vi "Measurement UI.vi"() -> ()   [LabVIEW 2021, in "Frequency Response_Audio ADC_UI.lvlib"]
uses:
  Frequency Response_Audio ADC_UI.lvlib
  shared/Audio ADC Shared.lvlib
panel:
  in  "MeasGraphs":T1(tab)
  out "FrequencyResponseGraph":cluster{"X":dbl[], "Y":dbl[]}(graph) caption="AC"
  out "RMSLevelGraph":cluster{"X":dbl[], "Y":dbl[]}(graph) caption="AC"
  out "THDResponseGraph":cluster{"X":dbl[], "Y":dbl[]}(graph) caption="AC"
  out "THD+NResponseGraph":cluster{"X":dbl[], "Y":dbl[]}(graph) caption="AC"
  out "TimeDomainGraph":cluster{dbl, "dt":dbl, "Time domain":dbl[]}[](graph) caption="AC"
  in  "Bit clock edge sync":u32=1
  in  "Frame sync pulse width":u32=32
  in  "Frame length":u32=64
  in  "Data justification":u32 caption="Data Justification"
  in  "Endianness":u32
  in  "Channel 0 offset":u32=1
  in  "Bit depth":u32=24
  in  "Channel length":u32=32
  in  "Channel count per frame":u32=2
  in  "Frame sync edge for channel 0":u32=1
  out "Time domain plot sizes":i32[](array[numeric])
  out "THD+N response":dbl[](array[numeric])
  out "Frequency response":dbl[](array[numeric])
  out "Time domain":dbl[](array[numeric])
  out "dt":dbl
  out "RMS levels":dbl[](array[numeric])
  out "THD response":dbl[](array[numeric])
  out "Frequency steps":dbl[](array[numeric])
  in  "Configure Protocol Settings":bool
  in  "Analog source resource name":string(combo) caption="RESOURCE NAME"
  in  "Protocol capture resource name":string(combo) caption="RESOURCE NAME"
  in  "Data line":u32 caption="DATA LINE"
  in  "Channel":u32 caption="CHANNEL"
  in  "MeasSettingsOptions":i32(listbox)=-1
  in  "Settling time":dbl caption="SETTLING TIME" format="%#_6ps"
  in  "Settling cycles":i32 caption="SETTLING CYCLES"
  in  "Maximum harmonic":i32=5 caption="MAX HARMONIC"
  in  "DC Offset":dbl caption="DC OFFSET" format="%#_6pV"
  out "Protocol settings":string="Protocol settings"
  in  "Sample rate":dbl=44100.0 caption="SAMPLE RATE" format="%#.6pHz"
  in  "Frequency spacing":string(combo)="Logarithmic" caption="FREQUENCY SPACING"
  in  "Measurement duration":dbl=0.001 caption="MEASUREMENT DURATION" format="%#_6ps"
  in  "Measurement cycles":i32=10 caption="MEASUREMENT CYCLES"
  in  "Frequency steps":i32=20 caption="FREQUENCY STEPS"
  out "Analog source":string="Analog source "
  in  "Amplitude":dbl=-1.0 caption="AMPLITUDE" format="%#_6pdB"
  in  "Full scale range":dbl=2.825 caption="FULL SCALE RANGE" format="%.3pV"
  in  "Frequency stop":dbl=10000.0 caption="FREQUENCY STOP" format="%#_6pHz"
  in  "Frequency start":dbl=100.0 caption="FREQUENCY START" format="%#_6pHz"
  out "Measurement settings":string="Measurement settings"
  in  "MeasSettings":bool
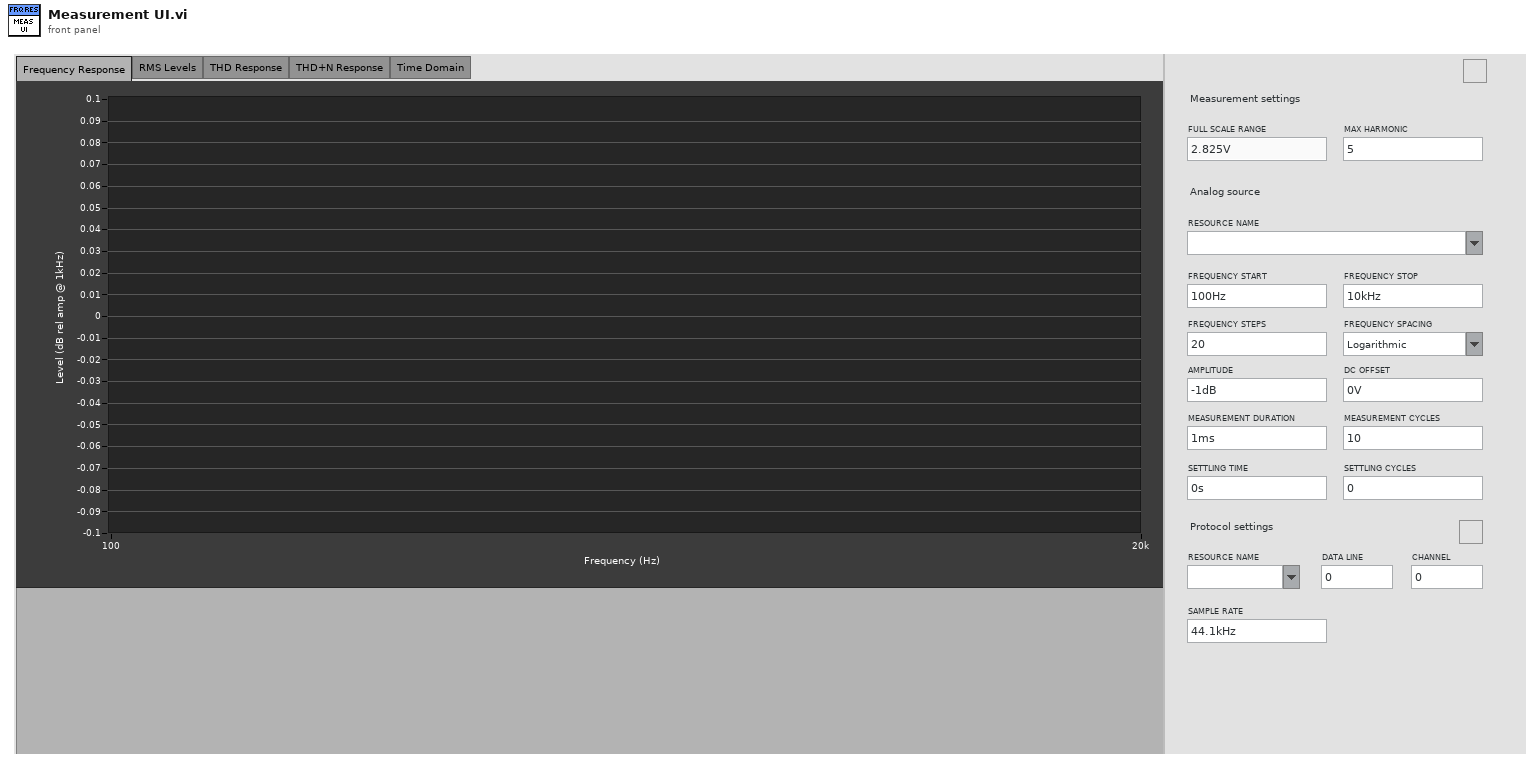
[diagram p1: front panel]
types:
  T1 = enum32{"Frequency Response", "RMS Levels", "THD Response", "THD+N Response", "Time Domain", "Hidden Controls"}
  T2 = enum16{"open", "replace", "create", "open or create", "replace or create", "replace or create with confirmation"}
  T3 = typedef "PDM Shared.lvlib/PCM Frame Sync Control.ctl" = cluster{"Frame Length":u16, "Frame Sync Pulse Width":u16, "Bit Clock Edge  Sync":T4}
  T4 = typedef "PDM Shared.lvlib/Digital Edge.ctl" = enum8{"Rising", "Falling"}
  T5 = typedef "PDM Shared.lvlib/PCM Data Format Configuration.ctl" = cluster{"Frame Sync Edge for Channel 0":T4, "Channel Count Per Frame":u8, "Channel Length":u16, "Bit Depth":u8, "Channel 0 Offset":u16, "Endianness":T6, "Data Justification":T7}
  T6 = typedef "PDM Shared.lvlib/PCM Bit Endianness.ctl" = enum16{"MSB First", "LSB First"}
  T7 = typedef "PDM Shared.lvlib/PCM Data Justification.ctl" = enum16{"Left Justified", "Right Justified"}
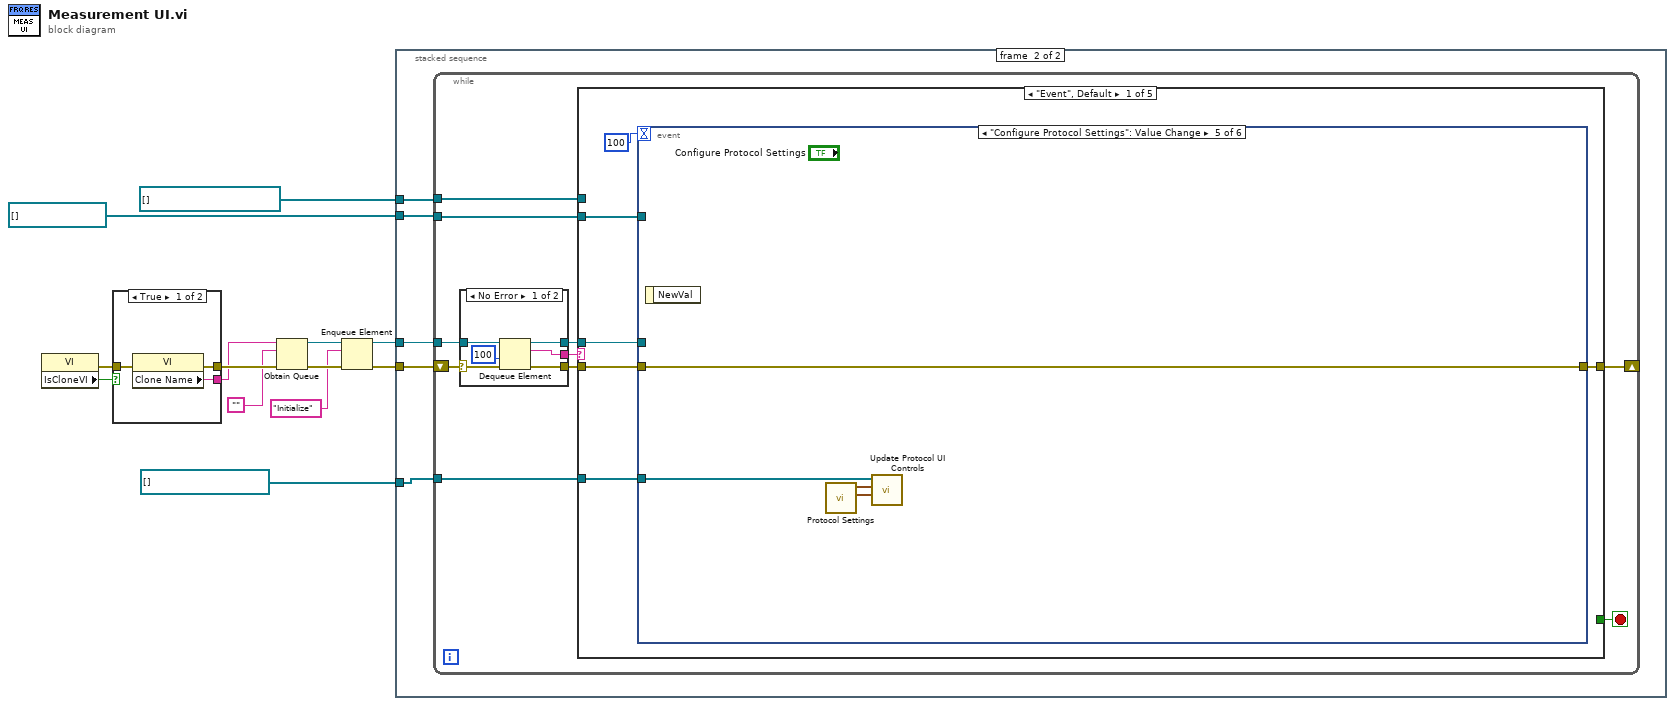
[diagram p0: block diagram]
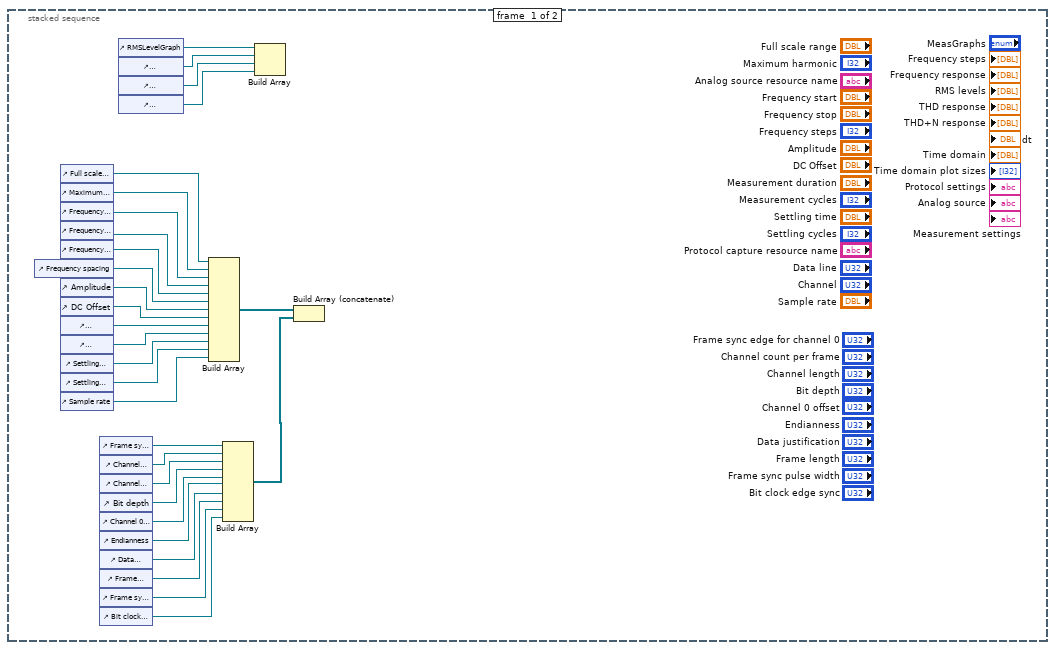
[diagram p2: hidden frame]
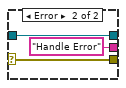
[diagram p3: hidden frame]
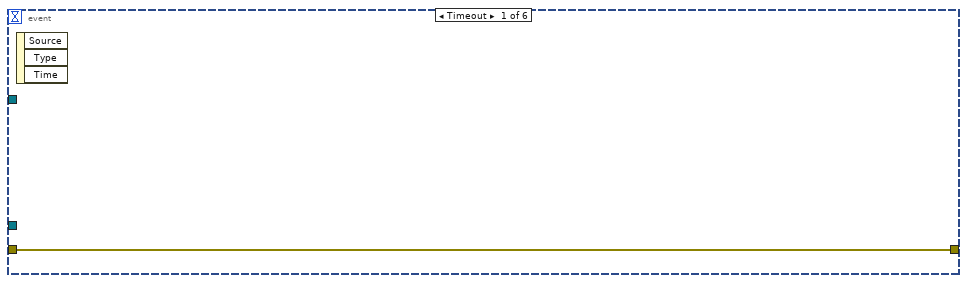
[diagram p4: hidden frame]
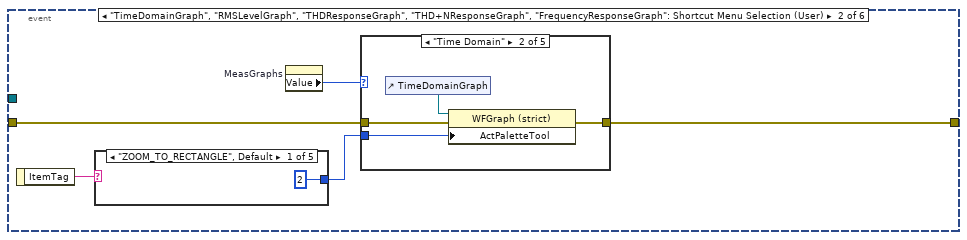
[diagram p5: hidden frame]
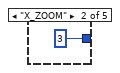
[diagram p6: hidden frame]
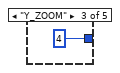
[diagram p7: hidden frame]
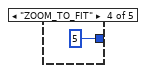
[diagram p8: hidden frame]
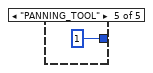
[diagram p9: hidden frame]
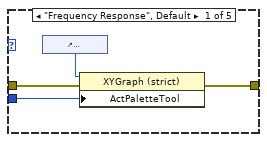
[diagram p10: hidden frame]
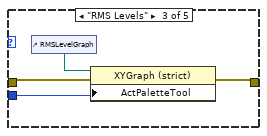
[diagram p11: hidden frame]
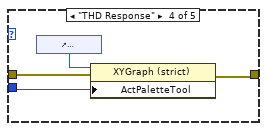
[diagram p12: hidden frame]
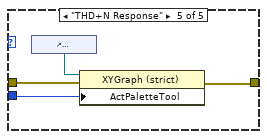
[diagram p13: hidden frame]
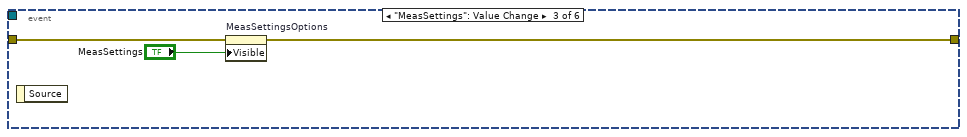
[diagram p14: hidden frame]
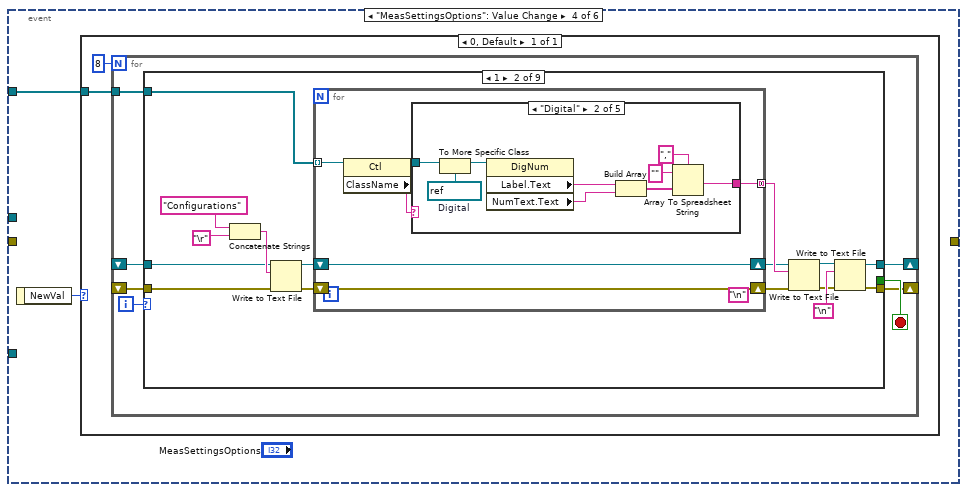
[diagram p15: hidden frame]
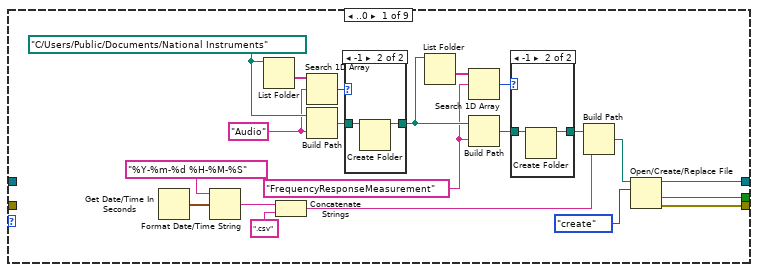
[diagram p16: hidden frame]
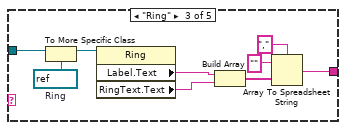
[diagram p20: hidden frame]
diagram:
  n1 = property class="VI"() -> (error out=w4:errorcluster, "IsCloneVI"=w5:bool)  [unwired: 2 in, 1 out]
  n2 = case shown="True" w5 {
    tunnel: [w16 w19] -> w13
    tunnel: [w15 w18] -> w12
    tunnel: w4 -> [w14 w17]
    frame True {
      n3 = property class="VI"(error in=w14) -> (error out=w16:errorcluster, "Clone Name"=w15:string)  [unwired: 1 in, 1 out]
    }
    frame False {
      n4 = property class="VI"(error in=w17) -> (error out=w19:errorcluster, "Name"=w18:string)  [unwired: 1 in, 1 out]
    }
  }
  n5 = Obtain Queue(name (unnamed)=w12, element data type="", error in (no error)=w13) -> (queue out=w9:refnum<queue>, error out=w11:errorcluster)  [unwired: 2 in, 1 out]
  n6 = Enqueue Element(queue=w9, element="Initialize", error in (no error)=w11) -> (queue out=w8:refnum<queue>, error out=w10:errorcluster)  [unwired: 1 in, 1 out]
  n7 = stacked-sequence {
    tunnel: w10 -> [_ w53]
    tunnel: w8 -> [_ w52]
    tunnel: refnum<vi>[] [] -> [_ w51]
    tunnel: refnum<vi>[] [] -> [_ w50]
    tunnel: refnum<vi>[] [] -> [_ w49]
    frame #0 {
      n8 = control-ref of="Frequency spacing"() -> (w43:refnum<vi>)
      n9 = control-ref of="Full scale range"() -> (w48:refnum<vi>)
      n10 = control-ref of="Maximum harmonic"() -> (w47:refnum<vi>)
      n11 = control-ref of="Frequency start"() -> (w46:refnum<vi>)
      n12 = control-ref of="Frequency stop"() -> (w45:refnum<vi>)
      n13 = control-ref of="Frequency steps"() -> (w44:refnum<vi>)
      n14 = control-ref of="Amplitude"() -> (w37:refnum<vi>)
      n15 = control-ref of="DC Offset"() -> (w36:refnum<vi>)
      n16 = control-ref of="Measurement duration"() -> (w42:refnum<vi>)
      n17 = control-ref of="Measurement cycles"() -> (w41:refnum<vi>)
      n18 = control-ref of="Settling time"() -> (w40:refnum<vi>)
      n19 = control-ref of="Settling cycles"() -> (w39:refnum<vi>)
      n20 = control-ref of="Sample rate"() -> (w38:refnum<vi>)
      n21 = control-ref of="Frame sync edge for channel 0"() -> (w31:refnum<vi>)
      n22 = control-ref of="Channel count per frame"() -> (w30:refnum<vi>)
      n23 = control-ref of="Channel length"() -> (w29:refnum<vi>)
      n24 = control-ref of="Bit depth"() -> (w28:refnum<vi>)
      n25 = control-ref of="Channel 0 offset"() -> (w27:refnum<vi>)
      n26 = control-ref of="Endianness"() -> (w26:refnum<vi>)
      n27 = control-ref of="Data justification"() -> (w25:refnum<vi>)
      n28 = control-ref of="Frame length"() -> (w24:refnum<vi>)
      n29 = control-ref of="Frame sync pulse width"() -> (w23:refnum<vi>)
      n30 = control-ref of="Bit clock edge sync"() -> (w22:refnum<vi>)
      n31 = control-ref of="RMSLevelGraph"() -> (w35:refnum<vi>)
      n32 = control-ref of="THDResponseGraph"() -> (w34:refnum<vi>)
      n33 = control-ref of="THD+NResponseGraph"() -> (w33:refnum<vi>)
      n34 = control-ref of="FrequencyResponseGraph"() -> (w32:refnum<vi>)
      n35 = Build Array(w48, w47, w46, w45, w44, w43, w37, w36, w42, w41, w40, w39, w38) -> (w21:refnum<vi>[])
      n36 = Build Array(w31, w30, w29, w28, w27, w26, w25, w24, w23, w22) -> (w20:refnum<vi>[])
      n37 = Build Array(w35, w34, w33, w32) -> ()  [unwired: 1 out]
      n38 = Build Array (concatenate)(w21, w20) -> ()  [unwired: 1 out]
    }
    frame #1 {
      n39 = while {
        shift-right: [w58] -> _
        shift-left: w53 -> [w63]
        tunnel: w52 -> [w61]
        tunnel: w49 -> [w56]
        tunnel: w51 -> [w55]
        tunnel: w50 -> [w54]
        stop <- w57 stop-if-true
        n40 = case shown="No Error" w63 {
          selector: w63 -> [w69 w72]
          tunnel: [w68 w72] -> w62
          tunnel: w61 -> [w67 w71]
          tunnel: [w66 w71] -> w60
          tunnel: [w65 "Handle Error"] -> w59
          frame No Error {
            n41 = Dequeue Element(queue=w67, timeout in ms (-1)=100, error in (no error)=w69) -> (queue out=w66:refnum<queue>, element=w65:string, error out=w68:errorcluster)  [unwired: 1 out]
          }
          frame Error {
          }
        }
        n42 = case shown="\"Event\", Default" w59 {
          tunnel: w62 -> [w77 w395 w432 w459 w460]
          tunnel: w60 -> [w75 _ _ w457 _]
          tunnel: [w78 w395 w432 w454 w460] -> w58
          tunnel: [_ _ _ TRUE _] -> w57
          tunnel: w56 -> [_ _ w406 _ _]
          tunnel: w55 -> [w74 _ _ _ _]
          tunnel: w54 -> [w73 _ _ _ _]
          frame "Event", Default {
            n43 = event shown="[4] \"Configure Protocol Settings\": Value Change" {
              selector: _ -> [_ _ _ _ _ _]
              dyn-events: _ -> [_ _ _ _ _ _]
              timeout: 100 -> [_ _ _ _ _ _]
              tunnel: [w79 w80 w110 _ w382 w385] -> w78
              tunnel: w77 -> [w79 w82 w112 _ w382 w386]
              tunnel: w75 -> [_ _ _ _ _ w384]
              tunnel: w74 -> [_ _ _ _ w379 _]
              tunnel: w73 -> [_ _ _ w113 _ _]
              event Timeout {
                n44 = event-data() -> ()  [unwired: 1 in, 3 out]
              }
              event "TimeDomainGraph", "RMSLevelGraph", "THDResponseGraph", "THD+NResponseGraph", "FrequencyResponseGraph": Shortcut Menu Selection (User) {
                n45 = event-data() -> ("ItemTag"=w83:string)  [unwired: 1 in]
                n46 = case shown="\"ZOOM_TO_RECTANGLE\", Default" w83 {
                  tunnel: [2 3 4 5 1] -> w81
                  frame "ZOOM_TO_RECTANGLE", Default {
                  }
                  frame "X_ZOOM" {
                  }
                  frame "Y_ZOOM" {
                  }
                  frame "ZOOM_TO_FIT" {
                  }
                  frame "PANNING_TOOL" {
                  }
                }
                n47 = property on="MeasGraphs" class="TabCtl (strict)"() -> ("Value"=w84:T1)  [unwired: 2 in, 2 out]
                n48 = case shown="\"Time Domain\"" w84 {
                  tunnel: w82 -> [w93 w96 w100 w105 w109]
                  tunnel: w81 -> [w90 w95 w99 w102 w108]
                  tunnel: [w92 w94 w98 w104 w107] -> w80
                  frame "Frequency Response", Default {
                    n49 = control-ref of="FrequencyResponseGraph"() -> (w91:refnum<vi>)
                    n50 = property class="XYGraph (strict)"(reference=w91, error in=w93, "ActPaletteTool"=w90) -> (error out=w92:errorcluster)  [unwired: 1 out]
                  }
                  frame "Time Domain" {
                    n51 = control-ref of="TimeDomainGraph"() -> (w97:refnum<vi>)
                    n52 = property class="WFGraph (strict)"(reference=w97, error in=w96, "ActPaletteTool"=w95) -> (error out=w94:errorcluster)  [unwired: 1 out]
                  }
                  frame "RMS Levels" {
                    n53 = control-ref of="RMSLevelGraph"() -> (w101:refnum<vi>)
                    n54 = property class="XYGraph (strict)"(reference=w101, error in=w100, "ActPaletteTool"=w99) -> (error out=w98:errorcluster)  [unwired: 1 out]
                  }
                  frame "THD Response" {
                    n55 = control-ref of="THDResponseGraph"() -> (w103:refnum<vi>)
                    n56 = property class="XYGraph (strict)"(reference=w103, error in=w105, "ActPaletteTool"=w102) -> (error out=w104:errorcluster)  [unwired: 1 out]
                  }
                  frame "THD+N Response" {
                    n57 = control-ref of="THD+NResponseGraph"() -> (w106:refnum<vi>)
                    n58 = property class="XYGraph (strict)"(reference=w106, error in=w109, "ActPaletteTool"=w108) -> (error out=w107:errorcluster)  [unwired: 1 out]
                  }
                }
              }
              event "MeasSettings": Value Change {
                n59 = event-data() -> ()  [unwired: 1 in, 1 out]
                n60 = property on="MeasSettingsOptions" class="LstBox (strict)"(error in=w112, "Visible"="MeasSettings") -> (error out=w110:errorcluster)  [unwired: 1 in, 1 out]
              }
              event "MeasSettingsOptions": Value Change {
                n61 = event-data() -> ("NewVal"=w114:i32)  [unwired: 1 in]
                n62 = case shown="0, Default" w114 {
                  tunnel: w113 -> [w115]
                  frame 0, Default {
                    n63 = for {
                      N: 8 -> [_]
                      shift-right: [w121] -> _
                      shift-left: _ -> [w120]
                      shift-right: [w119] -> _
                      shift-left: _ -> [w118]
                      tunnel: w115 -> [w117]
                      i -> [w123]
                      stop <- w122 stop-if-true
                      n64 = case shown="1" w123 {
                        tunnel: [w137 _ _ _ _ _ _ _ _] -> w122
                        tunnel: [w143 w152 w216 w247 w279 w311 w341 refnum<file> refnum ("refnum out") w378] -> w121
                        tunnel: w120 -> [_ w163 w236 w268 w300 w332 w349 w376 w378]
                        tunnel: [w136 w153 w214 w245 w277 w309 w340 w374 w377] -> w119
                        tunnel: w118 -> [_ w161 w235 w267 w299 w331 w350 w373 w377]
                        tunnel: w117 -> [_ w151 _ _ _ _ _ _ _]
                        frame ..0 {
                          w132 = "FrequencyResponseMeasurement" ("prompt")
                          w139 = "Audio" ("prompt")
                          w142 = path "C:/Users/Public/Documents/National Instruments" ("base path")
                          n65 = Get Date/Time In Seconds() -> (seconds since 1Jan1904=w129:timestamp)
                          n66 = Format Date/Time String(time format string (%c)="%Y-%m-%d %H-%M-%S", seconds (now)=w129) -> (date/time string=w128:string)  [unwired: 1 in]
                          n67 = List Folder(path=w142) -> (folder names=w140:string[])  [unwired: 3 in, 3 out]
                          n68 = Concatenate Strings(w128, ".csv" ("string")) -> (w125:string)
                          n69 = Search 1D Array(1D array=w140, element=w139) -> (index of element=w138:i32)  [unwired: 1 in]
                          n70 = Build Path(base path=w142, name or relative path=w139) -> (appended path=w141:path)
                          n71 = case shown="-1" w138 {
                            tunnel: w141 -> [w148 w150]
                            tunnel: [w148 w149] -> w133
                            frame Default {
                            }
                            frame -1 {
                              n72 = Create Folder(path (use dialog)=w150) -> (created path=w149:path)  [unwired: 2 in, 2 out]
                            }
                          }
                          n73 = List Folder(path=w133) -> (folder names=w135:string[])  [unwired: 3 in, 3 out]
                          n74 = Search 1D Array(1D array=w135, element=w132) -> (index of element=w134:i32)  [unwired: 1 in]
                          n75 = Build Path(base path=w133, name or relative path=w132) -> (appended path=w131:path)
                          n76 = case shown="-1" w134 {
                            tunnel: w131 -> [w145 w147]
                            tunnel: [w145 w146] -> w126
                            frame Default {
                            }
                            frame -1 {
                              n77 = Create Folder(path (use dialog)=w147) -> (created path=w146:path)  [unwired: 2 in, 2 out]
                            }
                          }
                          n78 = Build Path(base path=w126, name or relative path=w125) -> (appended path=w124:path)
                          n79 = Open/Create/Replace File(file path (use dialog)=w124, operation (0:open)=T2."create") -> (refnum out=w143:refnum<file>, cancelled=w137:bool, error out=w136:errorcluster)  [unwired: 4 in]
                        }
                        frame 1 {
                          (unwired) "\n"
                          n80 = Concatenate Strings("Configurations" ("format string"), "\r") -> (w164:string)
                          n81 = Write to Text File(file (use dialog)=w163, text=w164, error in=w161) -> (refnum out=w160:refnum<file>, error out=w162:errorcluster)  [unwired: 1 in, 1 out]
                          n82 = for {
                            shift-right: [w172] -> w158
                            shift-left: w160 -> [w172]
                            shift-right: [w171] -> w157
                            shift-left: w162 -> [w171]
                            tunnel: [w170] -> w159 mode=concatenating
                            tunnel: w151 -> [w167] mode=indexing
                            n83 = property class="Ctl"(reference=w167) -> (reference out=w169:refnum<vi>, "ClassName"=w168:string)  [unwired: 1 in, 1 out]
                            n84 = case shown="\"Digital\"" w168 {
                              tunnel: [_ w176 w186 w195 w204] -> w170
                              tunnel: w169 -> [_ w174 w184 w199 w208]
                              frame Default {
                              }
                              frame "Digital" {
                                w173 = refnum<vi> refnum  # Digital
                                n85 = To More Specific Class(target class=w173, reference=w174) -> (specific class reference=w175:refnum<vi>)  [unwired: 1 in, 1 out]
                                n86 = property class="DigNum"(reference=w175) -> ("Label.Text"=w181:string, "NumText.Text"=w180:string)  [unwired: 1 in, 2 out]
                                n87 = Build Array(w181, w180) -> (w177:string[])
                                n88 = Array To Spreadsheet String(delimiter (Tab)=",", array=w177, 3:"" ("format string")) -> (spreadsheet string=w176:string)
                              }
                              frame "Ring" {
                                w183 = refnum<vi> refnum  # Ring
                                n89 = To More Specific Class(target class=w183, reference=w184) -> (specific class reference=w185:refnum<vi>)  [unwired: 1 in, 1 out]
                                n90 = property class="Ring"(reference=w185) -> ("Label.Text"=w182:string, "RingText.Text"=w190:string)  [unwired: 1 in, 2 out]
                                n91 = Build Array(w182, w190) -> (w187:string[])
                                n92 = Array To Spreadsheet String(delimiter (Tab)=",", array=w187, 3:"" ("format string")) -> (spreadsheet string=w186:string)
                              }
                              frame "Enum" {
                                w198 = refnum<vi> refnum  # Enum
                                n93 = To More Specific Class(target class=w198, reference=w199) -> (specific class reference=w194:refnum<vi>)  [unwired: 1 in, 1 out]
                                n94 = property class="Enum"(reference=w194) -> ("Label.Text"=w193:string, "RingText.Text"=w192:string)  [unwired: 1 in, 2 out]
                                n95 = Build Array(w193, w192) -> (w191:string[])
                                n96 = Array To Spreadsheet String(delimiter (Tab)=",", array=w191, 3:"" ("format string")) -> (spreadsheet string=w195:string)
                              }
                              frame "ComboBox" {
                                w207 = refnum<vi> refnum  # ComboBox
                                n97 = To More Specific Class(target class=w207, reference=w208) -> (specific class reference=w203:refnum<vi>)  [unwired: 1 in, 1 out]
                                n98 = property class="CmbBox"(reference=w203) -> ("Label.Text"=w202:string, "Value"=w201:string)  [unwired: 1 in, 2 out]
                                n99 = Build Array(w202, w201) -> (w200:string[])
                                n100 = Array To Spreadsheet String(delimiter (Tab)=",", array=w200, 3:"" ("format string")) -> (spreadsheet string=w204:string)
                              }
                            }
                          }
                          n101 = Write to Text File(file (use dialog)=w158, text=w159, error in=w157) -> (refnum out=w155:refnum<file>, error out=w154:errorcluster)  [unwired: 1 in, 1 out]
                          n102 = Write to Text File(file (use dialog)=w155, text="\n", error in=w154) -> (refnum out=w152:refnum<file>, error out=w153:errorcluster)  [unwired: 1 in, 1 out]
                        }
                        frame 2 {
                          w209 = "\r"
                          n103 = property on="FrequencyResponseGraph" class="XYGraph (strict)"() -> ("Value"=w211:cluster{"X":dbl[], "Y":dbl[]})  [unwired: 2 in, 2 out]
                          n104 = Concatenate Strings("Results" ("string"), w209, "Frequency Response" ("string"), w209) -> (w233:string)
                          n105 = Write to Text File(file (use dialog)=w236, text=w233, error in=w235) -> (refnum out=w229:refnum<file>, error out=w228:errorcluster)  [unwired: 1 in, 1 out]
                          n106 = Build Array("Frequency (Hz)", "Level (dB rel amp @ 1kHz)") -> (w232:string[])
                          n107 = Unbundle By Name(w211) -> ("X"=w220:dbl[], "Y"=w221:dbl[])
                          n108 = Array To Spreadsheet String(delimiter (Tab)=",", array=w232, 3:"" ("format string")) -> (spreadsheet string=w227:string)
                          n109 = for {
                            tunnel: w220 -> [w241] mode=indexing
                            tunnel: w221 -> [w237] mode=indexing
                            tunnel: [w238] -> w222 mode=indexing
                            n110 = Format Into String(w241) -> (resulting string=w239:string)  [unwired: 3 in, 1 out]
                            n111 = Format Into String(w237) -> (resulting string=w240:string)  [unwired: 3 in, 1 out]
                            n112 = Build Array(w239, w240) -> (w238:string[])
                          }
                          n113 = Write to Text File(file (use dialog)=w229, text=w227, error in=w228) -> (refnum out=w226:refnum<file>, error out=w225:errorcluster)  [unwired: 1 in, 1 out]
                          n114 = Array To Spreadsheet String(delimiter (Tab)=",", array=w222, 3:"" ("format string")) -> (spreadsheet string=w219:string)
                          n115 = Write to Text File(file (use dialog)=w226, text=w219, error in=w225) -> (refnum out=w218:refnum<file>, error out=w217:errorcluster)  [unwired: 1 in, 1 out]
                          n116 = Write to Text File(file (use dialog)=w218, text="\n", error in=w217) -> (refnum out=w216:refnum<file>, error out=w214:errorcluster)  [unwired: 1 in, 1 out]
                        }
                        frame 3 {
                          n117 = property on="RMSLevelGraph" class="XYGraph (strict)"() -> ("Value"=w242:cluster{"X":dbl[], "Y":dbl[]})  [unwired: 2 in, 2 out]
                          n118 = Concatenate Strings("RMS Level" ("string"), "\r") -> (w265:string)
                          n119 = Build Array("Frequency (Hz)", "Level (Vrms)") -> (w264:string[])
                          n120 = Write to Text File(file (use dialog)=w268, text=w265, error in=w267) -> (refnum out=w261:refnum<file>, error out=w260:errorcluster)  [unwired: 1 in, 1 out]
                          n121 = Array To Spreadsheet String(delimiter (Tab)=",", array=w264, 3:"" ("format string")) -> (spreadsheet string=w259:string)
                          n122 = Unbundle By Name(w242) -> ("X"=w252:dbl[], "Y"=w253:dbl[])
                          n123 = Write to Text File(file (use dialog)=w261, text=w259, error in=w260) -> (refnum out=w258:refnum<file>, error out=w257:errorcluster)  [unwired: 1 in, 1 out]
                          n124 = for {
                            tunnel: w252 -> [w273] mode=indexing
                            tunnel: w253 -> [w269] mode=indexing
                            tunnel: [w270] -> w254 mode=indexing
                            n125 = Format Into String(w273) -> (resulting string=w271:string)  [unwired: 3 in, 1 out]
                            n126 = Format Into String(w269) -> (resulting string=w272:string)  [unwired: 3 in, 1 out]
                            n127 = Build Array(w271, w272) -> (w270:string[])
                          }
                          n128 = Array To Spreadsheet String(delimiter (Tab)=",", array=w254, 3:"" ("format string")) -> (spreadsheet string=w251:string)
                          n129 = Write to Text File(file (use dialog)=w258, text=w251, error in=w257) -> (refnum out=w249:refnum<file>, error out=w248:errorcluster)  [unwired: 1 in, 1 out]
                          n130 = Write to Text File(file (use dialog)=w249, text="\n", error in=w248) -> (refnum out=w247:refnum<file>, error out=w245:errorcluster)  [unwired: 1 in, 1 out]
                        }
                        frame 4 {
                          n131 = Concatenate Strings("THD Response" ("string"), "\r") -> (w297:string)
                          n132 = property on="THDResponseGraph" class="XYGraph (strict)"() -> ("Value"=w274:cluster{"X":dbl[], "Y":dbl[]})  [unwired: 2 in, 2 out]
                          n133 = Build Array("Frequency (Hz)", "THD (dB)") -> (w296:string[])
                          n134 = Write to Text File(file (use dialog)=w300, text=w297, error in=w299) -> (refnum out=w293:refnum<file>, error out=w292:errorcluster)  [unwired: 1 in, 1 out]
                          n135 = Array To Spreadsheet String(delimiter (Tab)=",", array=w296, 3:"" ("format string")) -> (spreadsheet string=w291:string)
                          n136 = Unbundle By Name(w274) -> ("X"=w284:dbl[], "Y"=w285:dbl[])
                          n137 = Write to Text File(file (use dialog)=w293, text=w291, error in=w292) -> (refnum out=w290:refnum<file>, error out=w289:errorcluster)  [unwired: 1 in, 1 out]
                          n138 = for {
                            tunnel: w284 -> [w305] mode=indexing
                            tunnel: w285 -> [w301] mode=indexing
                            tunnel: [w302] -> w286 mode=indexing
                            n139 = Format Into String(w305) -> (resulting string=w303:string)  [unwired: 3 in, 1 out]
                            n140 = Format Into String(w301) -> (resulting string=w304:string)  [unwired: 3 in, 1 out]
                            n141 = Build Array(w303, w304) -> (w302:string[])
                          }
                          n142 = Array To Spreadsheet String(delimiter (Tab)=",", array=w286, 3:"" ("format string")) -> (spreadsheet string=w283:string)
                          n143 = Write to Text File(file (use dialog)=w290, text=w283, error in=w289) -> (refnum out=w281:refnum<file>, error out=w280:errorcluster)  [unwired: 1 in, 1 out]
                          n144 = Write to Text File(file (use dialog)=w281, text="\n", error in=w280) -> (refnum out=w279:refnum<file>, error out=w277:errorcluster)  [unwired: 1 in, 1 out]
                        }
                        frame 5 {
                          n145 = property on="THD+NResponseGraph" class="XYGraph (strict)"() -> ("Value"=w306:cluster{"X":dbl[], "Y":dbl[]})  [unwired: 2 in, 2 out]
                          n146 = Concatenate Strings("THD+N Response" ("string"), "\r") -> (w329:string)
                          n147 = Build Array("Frequency (Hz)", "THD+N (dB)") -> (w328:string[])
                          n148 = Write to Text File(file (use dialog)=w332, text=w329, error in=w331) -> (refnum out=w325:refnum<file>, error out=w324:errorcluster)  [unwired: 1 in, 1 out]
                          n149 = Array To Spreadsheet String(delimiter (Tab)=",", array=w328, 3:"" ("format string")) -> (spreadsheet string=w323:string)
                          n150 = Unbundle By Name(w306) -> ("X"=w316:dbl[], "Y"=w317:dbl[])
                          n151 = Write to Text File(file (use dialog)=w325, text=w323, error in=w324) -> (refnum out=w322:refnum<file>, error out=w321:errorcluster)  [unwired: 1 in, 1 out]
                          n152 = for {
                            tunnel: w316 -> [w337] mode=indexing
                            tunnel: w317 -> [w333] mode=indexing
                            tunnel: [w334] -> w318 mode=indexing
                            n153 = Format Into String(w337) -> (resulting string=w335:string)  [unwired: 3 in, 1 out]
                            n154 = Format Into String(w333) -> (resulting string=w336:string)  [unwired: 3 in, 1 out]
                            n155 = Build Array(w335, w336) -> (w334:string[])
                          }
                          n156 = Array To Spreadsheet String(delimiter (Tab)=",", array=w318, 3:"" ("format string")) -> (spreadsheet string=w315:string)
                          n157 = Write to Text File(file (use dialog)=w322, text=w315, error in=w321) -> (refnum out=w313:refnum<file>, error out=w312:errorcluster)  [unwired: 1 in, 1 out]
                          n158 = Write to Text File(file (use dialog)=w313, text="\n", error in=w312) -> (refnum out=w311:refnum<file>, error out=w309:errorcluster)  [unwired: 1 in, 1 out]
                        }
                        frame 6 {
                          n159 = Concatenate Strings("Time Domain" ("string"), "\r") -> (w362:string)
                          n160 = Write to Text File(file (use dialog)=w349, text=w362, error in=w350) -> (refnum out=w359:refnum<file>, error out=w358:errorcluster)  [unwired: 1 in, 1 out]
                          n161 = Build Array("Time (s)", "Amplitude (V)") -> (w361:string[])
                          n162 = property on="dt" class="DigNum (strict)"() -> ("Value"=w338:dbl)  [unwired: 2 in, 2 out]
                          n163 = property on="Time domain" class="Arr (strict)"() -> ("Value"=w339:dbl[])  [unwired: 2 in, 2 out]
                          n164 = Array To Spreadsheet String(delimiter (Tab)=",", array=w361, 3:"" ("format string")) -> (spreadsheet string=w357:string)
                          n165 = Write to Text File(file (use dialog)=w359, text=w357, error in=w358) -> (refnum out=w356:refnum<file>, error out=w355:errorcluster)  [unwired: 1 in, 1 out]
                          n166 = for {
                            tunnel: [w368] -> w352 mode=indexing
                            tunnel: w339 -> [w367] mode=indexing
                            tunnel: w338 -> [w365]
                            i -> [w366]
                            n167 = Multiply(x=w365, y=w366) -> (x*y=w364:dbl)
                            n168 = Format Into String(w364) -> (resulting string=w369:string)  [unwired: 3 in, 1 out]
                            n169 = Format Into String(w367) -> (resulting string=w370:string)  [unwired: 3 in, 1 out]
                            n170 = Build Array(w369, w370) -> (w368:string[])
                          }
                          n171 = Array To Spreadsheet String(delimiter (Tab)=",", array=w352, 3:"" ("format string")) -> (spreadsheet string=w351:string)
                          n172 = Write to Text File(file (use dialog)=w356, text=w351, error in=w355) -> (refnum out=w343:refnum<file>, error out=w342:errorcluster)  [unwired: 1 in, 1 out]
                          n173 = Write to Text File(file (use dialog)=w343, text="\n", error in=w342) -> (refnum out=w341:refnum<file>, error out=w340:errorcluster)  [unwired: 1 in, 1 out]
                        }
                        frame 7 {
                          w372 = FALSE ("Visible")
                          n174 = Close File(refnum=w376, error in=w373) -> (error out=w374:errorcluster)  [unwired: 1 out]
                          n175 = property on="MeasSettingsOptions" class="LstBox (strict)"("Visible"=w372, "Value"=-1 ("MeasSettingsOptions")) -> ()  [unwired: 2 in, 2 out]
                          n176 = property on="MeasSettings" class="Bool (strict)"("Value"=w372) -> ()  [unwired: 2 in, 2 out]
                        }
                        frame Default {
                        }
                      }
                    }
                  }
                }
              }
              event "Configure Protocol Settings": Value Change {
                n177 = event-data() -> ()  [unwired: 1 in, 1 out]
                n178 = call "Protocol Settings.vi"() -> ("Frame sync clock control"=w380:T3, "PDM data configuration"=w381:T5)  [unwired: 10 in]
                n179 = call "Update Protocol UI Controls.vi"("Frame Sync Clock Control"=w380, "PCM Data Configuration"=w381, "Control references"=w379) -> ()  [unwired: 9 in]
              }
              event Panel Close? {
                n180 = event-data() -> ()  [unwired: 1 in, 4 out]
                n181 = Enqueue Element(queue=w384, element="Exit", error in (no error)=w386) -> (error out=w385:errorcluster)  [unwired: 1 in, 2 out]
                n182 = event-data("Discard?"=TRUE) -> ()  [unwired: 1 in, 1 out]
              }
            }
          }
          frame "Initialize" {
            w388 = 2 ("Palette:Active Tool")
            n183 = control-ref of="TimeDomainGraph"() -> (w390:refnum<vi>)
            n184 = control-ref of="FrequencyResponseGraph"() -> (w391:refnum<vi>)
            n185 = control-ref of="THDResponseGraph"() -> (w393:refnum<vi>)
            n186 = control-ref of="RMSLevelGraph"() -> (w392:refnum<vi>)
            n187 = control-ref of="THD+NResponseGraph"() -> (w389:refnum<vi>)
            n188 = Build Array(w391, w393, w392, w389) -> (w394:refnum<vi>[])
            n189 = for {
              tunnel: w394 -> [w404] mode=indexing
              tunnel: w388 -> [w403]
              n190 = property class="XYGraph (strict)"(reference=w404, "ActPaletteTool"=w403) -> ()  [unwired: 1 in, 2 out]
            }
            n191 = stacked-sequence {
              frame #0 {
                n192 = call "Detected DSGs.vi"() -> ("AO channels"=w398:string[])  [unwired: 11 in]
                n193 = Index Array(array=w398, index=0) -> (element=w397:string)
                n194 = property on="Analog source resource name" class="CmbBox"("Strings[]"=w398, "Value"=w397) -> ()  [unwired: 2 in, 2 out]
              }
              frame #1 {
                n195 = call "Detected PDMs.vi"() -> ("PDM devices"=w401:string[])  [unwired: 11 in]
                n196 = Index Array(array=w401, index=0) -> (element=w400:string)
                n197 = property on="Protocol capture resource name" class="CmbBox"("Strings[]"=w401, "Value"=w400) -> ()  [unwired: 2 in, 2 out]
              }
              frame #2 {
                n198 = property on="Frequency steps" class="DigNum (strict)"("Val(Sgnl)"=20 ("Value (Signaling)")) -> ()  [unwired: 2 in, 2 out]
              }
            }
            n199 = property class="WFGraph (strict)"(reference=w390, "ActPaletteTool"=w388) -> ()  [unwired: 1 in, 2 out]
          }
          frame "Post UI Update" {
            w411 = u32[] [15787074, 5682409, 15535092, 40563, 13983232, 35009, 15113984, 13400487, 15993633, 10221451, 8148942, 15869817, 32914, 10196480, 6271923, 16355671]  # Plot colors
            # "This case will be triggered, after framework updates the User interface with result values."
            n200 = local read "Time domain plot sizes"() -> (w413:i32[])
            n201 = property on="TimeDomainGraph" class="WFGraph (strict)"() -> ("Value"=w417:cluster{dbl, "dt":dbl, "Time domain":dbl[]}[])  [unwired: 2 in, 2 out]
            n202 = Not Equal?(x="Linear", y="Frequency spacing") -> (x != y?=w408:bool)
            n203 = Boolean To (0,1)(Boolean=w408) -> (0, 1=w405:i16)
            n204 = Array Size(array=w417) -> (size(s)=w415:i32)
            n205 = for {
              tunnel: w406 -> [w434] mode=indexing
              tunnel: w405 -> [w433]
              n206 = property class="XYGraph (strict)"(reference=w434, "XScale.Mapping Mode"=w433) -> ()  [unwired: 1 in, 2 out]
            }
            n207 = Array Size(array=w413) -> (size(s)=w416:i32)
            n208 = Not Equal?(x=w415, y=w416) -> (x != y?=w414:bool)
            n209 = case shown="True" w414 {
              tunnel: w413 -> [w435 w436]
              tunnel: [w435 w436] -> w412
              tunnel: w411 -> [_ w437]
              frame False {
              }
              frame True {
                n210 = for {
                  tunnel: w436 -> [_] mode=indexing
                  tunnel: w437 -> [w440]
                  i -> [w442]
                  n211 = Quotient & Remainder(x=w442, y=16) -> (x-y*floor(x/y)=w439:i32)  [unwired: 1 out]
                  n212 = Index Array(array=w440, index=w439) -> (element=w438:u32)
                  n213 = property on="TimeDomainGraph" class="WFGraph (strict)"("Active Plot"=w442, "Plot.Plot Color"=w438) -> ()  [unwired: 2 in, 2 out]
                }
              }
            }
            n214 = local read "Frequency response"() -> (w431:dbl[])
            n215 = local read "THD+N response"() -> (w424:dbl[])
            n216 = local read "Frequency steps"() -> (w429:dbl[])
            n217 = local read "THD response"() -> (w425:dbl[])
            n218 = local read "RMS levels"() -> (w422:dbl[])
            n219 = Bundle By Name(cluster=cluster{"X":dbl[], "Y":dbl[]} {"X"=[], "Y"=[]} ("THD vs Amplitude"), "X"=w429) -> (w421:cluster{"X":dbl[], "Y":dbl[]})
            n220 = Bundle By Name(cluster=w421, "Y"=w422) -> (→"RMSLevelGraph":cluster{"X":dbl[], "Y":dbl[]})
            n221 = local read "Time domain"() -> (w420:dbl[])
            n222 = Bundle By Name(cluster=w421, "Y"=w425) -> (→"THDResponseGraph":cluster{"X":dbl[], "Y":dbl[]})
            n223 = Bundle By Name(cluster=w421, "Y"=w424) -> (→"THD+NResponseGraph":cluster{"X":dbl[], "Y":dbl[]})
            n224 = local read "dt"() -> (w419:dbl)
            n225 = Bundle By Name(cluster=w421, "Y"=w431) -> (→"FrequencyResponseGraph":cluster{"X":dbl[], "Y":dbl[]})
            n226 = for {
              tunnel: w412 -> [w450] mode=indexing
              shift-right: [w446] -> _
              shift-left: w420 -> [w452]
              tunnel: w419 -> [w447]
              shift-right: [w449] -> _
              shift-left: 0 -> [w451]
              tunnel: [w445] -> w407 mode=indexing
              n227 = Multiply(x=w447, y=w451) -> (x*y=w448:dbl)
              n228 = Add(x=w451, y=w450) -> (x+y=w449:i32)
              n229 = Delete From Array(array=w452, length=w450, index=0) -> (deleted portion=w443:dbl[], array with subset deleted=w446:dbl[])
              n230 = Bundle(w448, "dt"=w447, "Time domain"=w443) -> (w445:cluster{dbl, "dt":dbl, "Time domain":dbl[]})  [unwired: 1 in]
            }
            "TimeDomainGraph" <- w407
          }
          frame "Exit" {
            # "This case is triggered to close the User Interface from framework"
            n231 = Flush Queue(queue=w457, error in (no error)=w459) -> (queue out=w456:refnum<queue>, error out=w455:errorcluster)  [unwired: 1 out]
            n232 = Release Queue(queue=w456, force destroy? (F)=TRUE, error in (no error)=w455) -> (error out=w454:errorcluster)  [unwired: 2 out]
          }
          frame "Handle Error" {
          }
        }
      }
    }
  }
